vi "AssertValueByArrayIndex.vi"(0 "VI Reference In":refnum<vi>, 1 "Test Label":string, 2 "delimiter (>>)":string=">>", 3 "Assert Only? (F)":bool, 5 "Control Path":string, 7 "Focus Item Index":i32[](array[numeric]), 11 "Error In":errorcluster, 12 "Assert Interval(10 ms)":u32=10, 13 "Timeout(5 sec)":dbl=5.0) -> (4 "VI Reference Out":refnum<vi>, 6 "Asserted Value":i32[](array[numeric]), 15 "Error Out":errorcluster)   [LabVIEW 2016, in "Drona.lvlib" / "AssertControlValue.lvlib" / "AssertMCListbox.lvlib"]
doc: "Asserts if the focus item index values of multi-select multi-column listbox control are equal.\n\nThe input control name is given as a string, incase of the path, use delimiters in between the path.\nThis VI gets the control value until the value is equal to the input value."
uses:
  AssertMCListbox.lvlib
  Get/GetControlRef/GetControlRefByPath.vi
  <vilib>/addons/_JKI Toolkits/Caraya/classes/Assert/Assert Equal Value_Variant.vi
  <vilib>/Utility/error.llb/Error Cluster From Error Code.vi
  <vilib>/ErrorRing/Error Ring.xnode
  <vilib>/addons/_JKI Toolkits/Caraya/classes/Assert/Assert.lvclass
  Get/GetControlRef/GetControlRef.lvlib
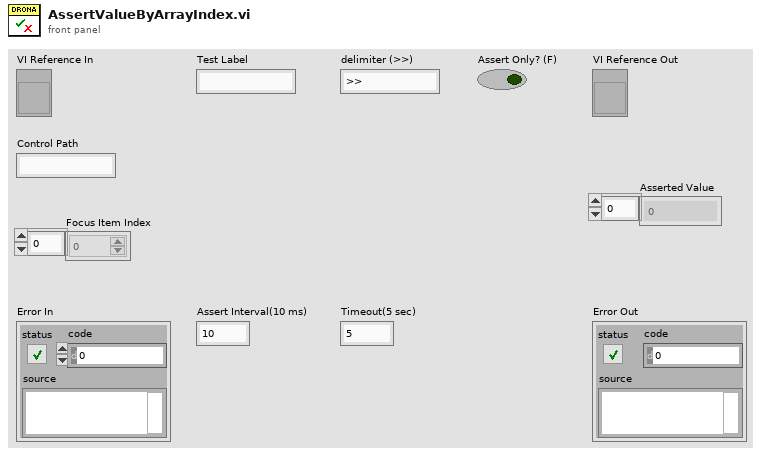
[diagram p1: front panel]
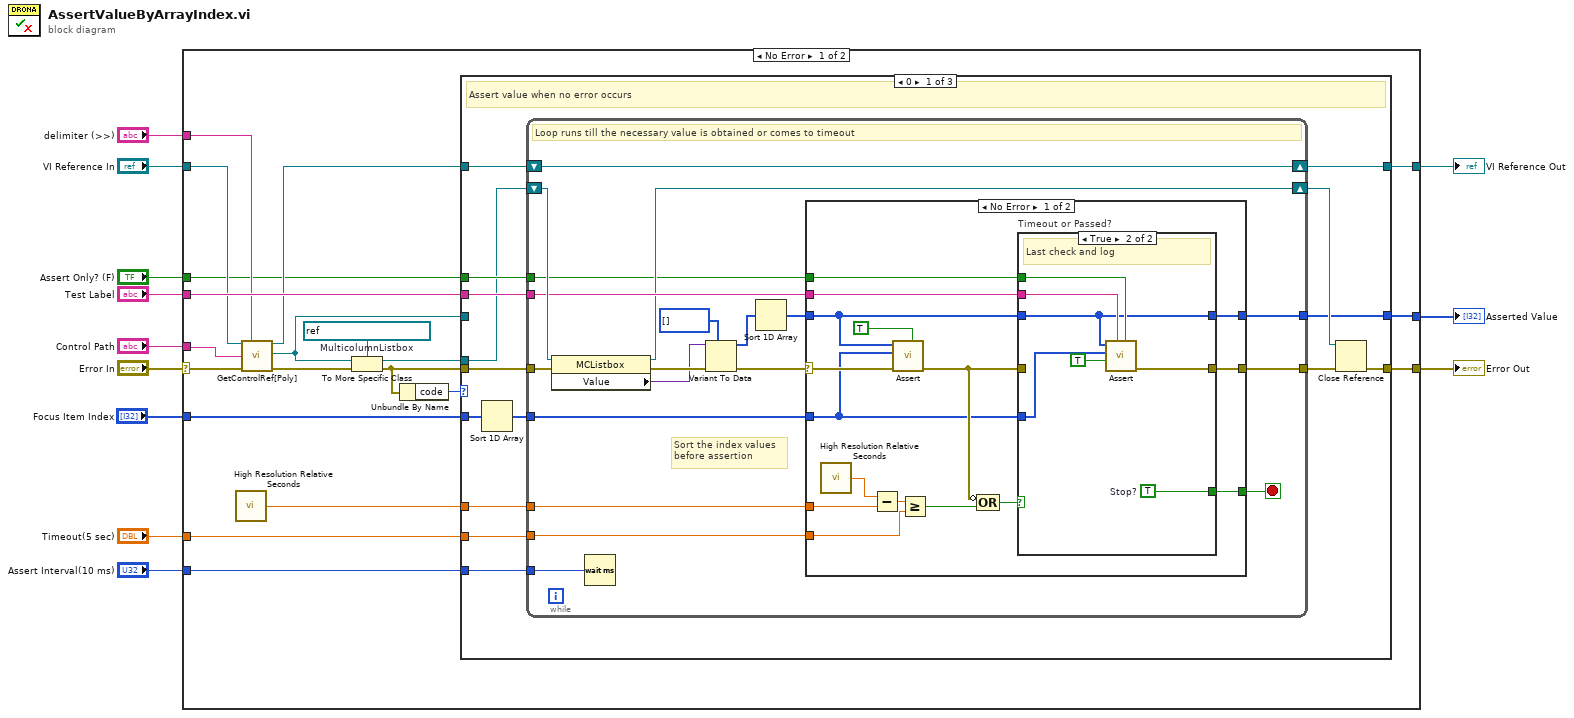
[diagram p0: block diagram]
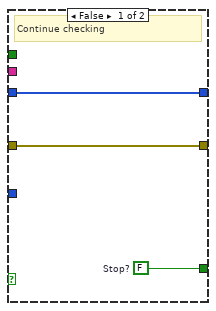
[diagram p2: hidden frame]
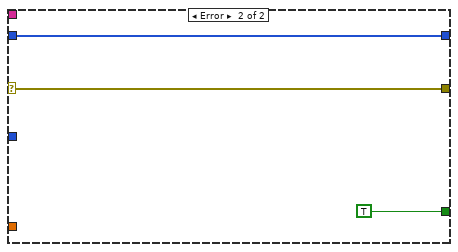
[diagram p3: hidden frame]
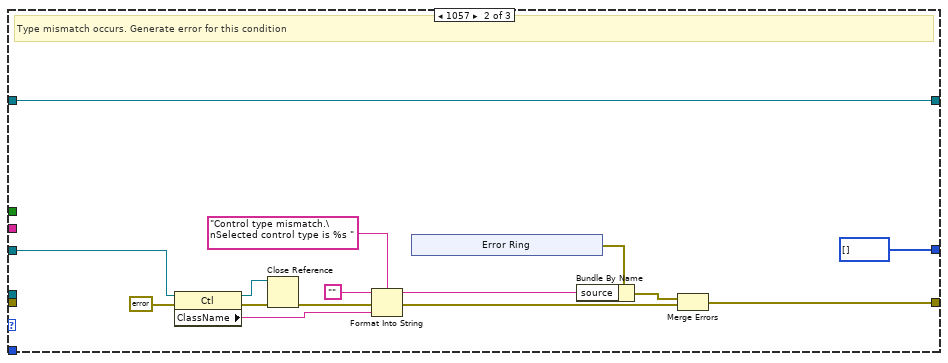
[diagram p4: hidden frame]
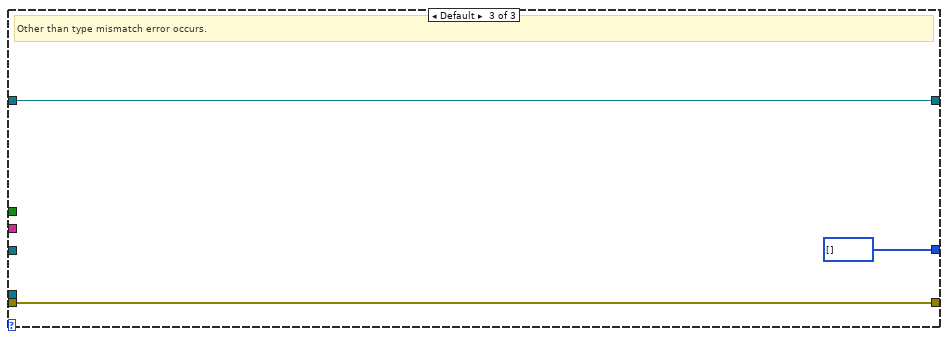
[diagram p5: hidden frame]
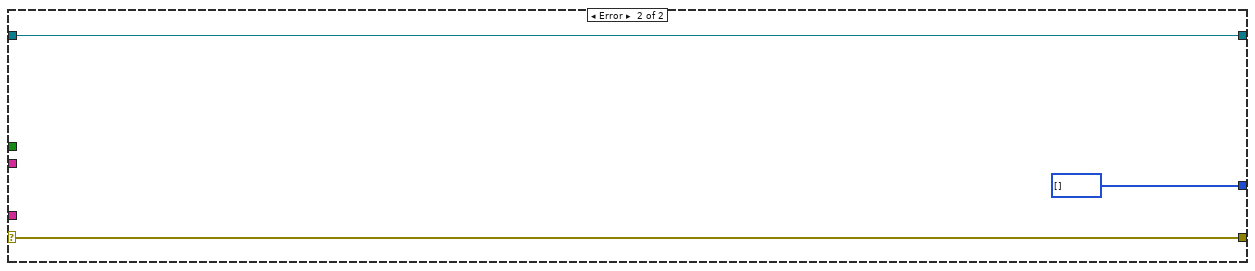
[diagram p6: hidden frame]
diagram:
  n1 = case shown="No Error" "Error In" {
    selector: "Error In" -> [w28 w121]
    tunnel: "Timeout(5 sec)" -> [w32 _]
    tunnel: [w31 w120] -> w11
    tunnel: "Focus Item Index" -> [w16 _]
    tunnel: [w22 w121] -> w10
    tunnel: "Assert Interval(10 ms)" -> [w30 _]
    tunnel: "Test Label" -> [w29 _]
    tunnel: "VI Reference In" -> [w27 w120]
    tunnel: "Control Path" -> [w26 _]
    tunnel: "delimiter (>>)" -> [w21 _]
    tunnel: "Assert Only? (F)" -> [w20 _]
    tunnel: [w19 i32[] []] -> w2
    frame No Error {
      w18 = refnum<vi> refnum  # MulticolumnListbox
      n2 = call <vilib>:"High Resolution Relative Seconds.vi"() -> ("relative seconds"=w25:dbl)
      n3 = call-poly "GetControlRef[Poly].vi"("VI Reference In"=w27, "delimiter (>>)"=w21, "Control Path"=w26, "error In"=w28) -> ("VI Reference Out"=w23:refnum<vi>, "Ctl Refnum"=w13:refnum<vi>, "error out"=w24:errorcluster)  [unwired: 9 in]
      n4 = To More Specific Class(target class=w18, reference=w13, error in=w24) -> (specific class reference=w17:refnum<vi>, error out=w15:errorcluster)
      n5 = Unbundle By Name(w15) -> ("code"=w14:i32)
      n6 = case shown="0" w14 {
        tunnel: w32 -> [w47 _ _]
        tunnel: [w46 w96 w116] -> w31
        tunnel: w30 -> [w44 _ _]
        tunnel: w29 -> [w43 _ _]
        tunnel: w25 -> [w42 _ _]
        tunnel: w23 -> [w41 w96 w116]
        tunnel: [w40 w99 w118] -> w22
        tunnel: w20 -> [w38 _ _]
        tunnel: [w37 i32[] [] i32[] []] -> w19
        tunnel: w15 -> [w36 _ w118]
        tunnel: w17 -> [w35 _ _]
        tunnel: w16 -> [w34 _ _]
        tunnel: w13 -> [_ w98 _]
        frame 0 {
          # "Assert value when no error occurs"
          n7 = Sort 1D Array(array=w34) -> (sorted array=w33:i32[])
          n8 = while {
            tunnel: w33 -> [w53]
            tunnel: w47 -> [w65]
            tunnel: w42 -> [w66]
            tunnel: w36 -> [w60]
            tunnel: [w63] -> w45
            tunnel: w44 -> [w61]
            tunnel: w43 -> [w57]
            shift-right: [w58] -> w46
            shift-left: w41 -> [w58]
            shift-right: [w56] -> w39
            shift-left: w35 -> [w59]
            tunnel: w38 -> [w55]
            tunnel: [w54] -> w37
            stop <- w64 stop-if-true
            # "Sort the index values \nbefore assertion"
            # "Loop runs till the necessary value is obtained or comes to timeout"
            n9 = property on="Property Node" class="MCListbox"(reference=w59, error in=w60) -> (reference out=w56:refnum<vi>, error out=w62:errorcluster, "Value"=w51:variant)
            n10 = Wait (ms)(milliseconds to wait=w61) -> ()  [unwired: 1 out]
            n11 = Variant To Data(error in=w62, type=i32[] [], Variant=w51) -> (data=w49:i32[], error out=w52:errorcluster)
            n12 = Sort 1D Array(array=w49) -> (sorted array=w48:i32[])
            n13 = case shown="No Error" w52 {
              selector: w52 -> [w78 w95]
              tunnel: w66 -> [w82 _]
              tunnel: w65 -> [w79 _]
              tunnel: [w69 TRUE] -> w64
              tunnel: [w70 w95] -> w63
              tunnel: w53 -> [w71 _]
              tunnel: w48 -> [w72 w93]
              tunnel: w57 -> [w77 _]
              tunnel: w55 -> [w68 _]
              tunnel: [w67 w93] -> w54
              frame No Error {
                n14 = call <vilib>:"High Resolution Relative Seconds.vi"() -> ("relative seconds"=w81:dbl)
                n15 = Subtract(x=w81, y=w82) -> (x-y=w80:dbl)
                n16 = call-poly <vilib>:"Assert.vi"("Assert Only? (F)"=TRUE, "error in (no error)"=w78, "Y"=w71, "X"=w72) -> ("error out"=w75:errorcluster)  [unwired: 7 in]
                n17 = Greater Or Equal?(x=w80, y=w79) -> (x >= y?=w76:bool)
                n18 = Compound Arithmetic op=OR(invert w75, w76) -> (w74:bool)
                n19 = case "Timeout or Passed?" shown="True" w74 {
                  tunnel: w75 -> [w85 _]
                  tunnel: w71 -> [_ w91]
                  tunnel: w72 -> [w83 w86]
                  tunnel: w77 -> [_ w92]
                  tunnel: [w85 w90] -> w70
                  tunnel: [w84 w89] -> w69
                  tunnel: w68 -> [_ w87]
                  tunnel: [w83 w86] -> w67
                  frame False {
                    w84 = FALSE  # Stop?
                    # "Continue checking"
                  }
                  frame True {
                    w89 = TRUE  # Stop?
                    # "Last check and log"
                    n20 = call-poly <vilib>:"Assert.vi"("Assert Only? (F)"=w87, "Label"=w92, "Register with caller test (F)"=TRUE, "Y"=w91, "X"=w86) -> ("error out"=w90:errorcluster)  [unwired: 6 in]
                  }
                }
              }
              frame Error {
              }
            }
          }
          n21 = Close Reference(reference=w39, error in (no error)=w45) -> (error out=w40:errorcluster)
        }
        frame 1057 {
          # "Type mismatch occurs. Generate error for this condition"
          n22 = property class="Ctl"(reference=w98, error in=errorcluster {"status"=FALSE, "code"=0, "source"=""} ("error out")) -> (reference out=w100:refnum<vi>, error out=w110:errorcluster, "ClassName"=w107:string)
          n23 = Close Reference(reference=w100, error in (no error)=w110) -> (error out=w101:errorcluster)
          n24 = Format Into String(format string="Control type mismatch.\nSelected control type is %s ", initial string="", error in=w101, w107) -> (resulting string=w104:string, error out=w102:errorcluster)
          n25 = xnode "Error Ring"() -> ("error out"=w105:errorcluster)
          n26 = Bundle By Name(cluster=w105, "source"=w104) -> (w103:errorcluster)
          n27 = Merge Errors(w103, w102) -> (w99:errorcluster)
        }
        frame Default {
          # "Other than type mismatch error occurs."
        }
      }
    }
    frame Error {
    }
  }
  "Error Out" <- w10
  "VI Reference Out" <- w11
  "Asserted Value" <- w2
